vi "Test.vi"() -> ()   [LabVIEW 2018]
uses:
  <vilib>/Platform/TimedLoop/XDataNode/timing_clust.ctl
  <vilib>/Platform/TimedLoop/XDataNode/nitl_modes.ctl
  <vilib>/Platform/TimedLoop/XDataNode/wakeup.ctl
  <vilib>/rvi/Emulation/niFpgaSctlEmulationGetInTimedLoop.vi
  <vilib>/rvi/Emulation/niFpgaEmulationReportErrorSimple.vi
  <vilib>/rvi/Emulation/niFpgaGetClockAttributes.vi
  <vilib>/rvi/Emulation/niFpgaCriticalErrorInLSC.vi
  <vilib>/rvi/eio/common/nirviEmuTemplateMethod_errors.vi
  <vilib>/Platform/TimedLoop/XDataNode/XDataNode.xnode
  <vilib>/eio/EIONode/EIONode.xnode
  <vilib>/Platform/TimedLoop/XDataNode/XDNodeRunTimeDep.lvlib
panel:
  out "Record":i16[](array[numeric])
  out "Round":u64 format="%.0e"
  out "Out":bool
  out "Test":bool
  out "2V":bool
  out "2H":bool
  out "1V":bool
  out "1H":bool
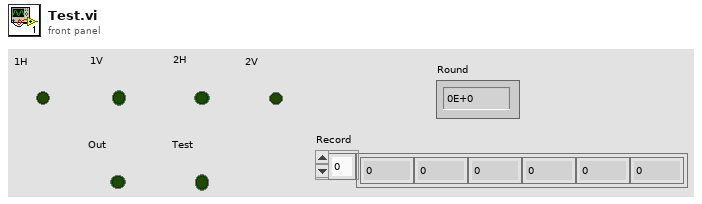
[diagram p1: front panel]
types:
  T1 = typedef "XDNodeRunTimeDep.lvlib/timing_clust.ctl" = cluster{"Expected End [f-1]":u64, "Actual End [f-1]":u64, "Finished Late? [f-1]":bool, "Expected End [i-1]":u64, "Actual End [i-1]":u64, "Finished Late? [i-1]":bool, "Expected Start [i]":u64, "Actual Start [i]":u64, "Expected Start [f]":u64, "Actual Start [f]":u64, "Source Name":string, "Structure Name":string, "Period":i64, "Deadline":i64, "Offset":i64, "Start":i64, "Priority":i32, "Timeout":i32, "Mode":T2, "Wakeup Reason":T3, "Error":errorcluster, "Source Type":string, "Secondary Source Type":string, "Global End Time":u64, "Global Start Time":u64, "Frame Duration":u64, "Iteration Duration":u64, "Assigned CPU":i32, "I/O Scan Engine Mode":u32}
  T2 = typedef "XDNodeRunTimeDep.lvlib/nitl_modes.ctl" = enum32{"No Change", "Process missed periods, maintain original phase", "Discard missed periods, maintain original phase", "Process missed periods, ignore original phase", "Discard missed periods, ignore original phase"}
  T3 = typedef "XDNodeRunTimeDep.lvlib/wakeup.ctl" = enum32{"Normal", "Aborted", "Asynchronous wakeup", "Timing source error", "Timed loop error", "Timeout"}
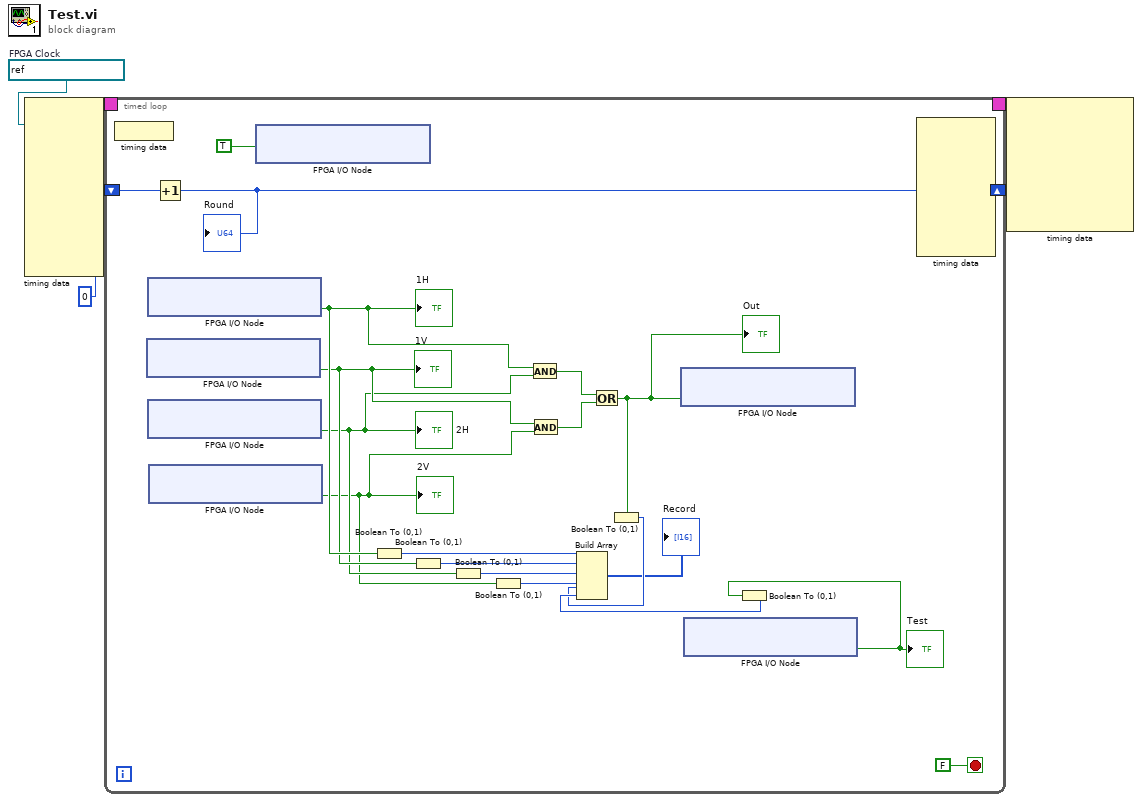
[diagram p0: block diagram]
diagram:
  w2 = refnum<k21> "200 MHz Clock"  # FPGA Clock
  n1 = node-c288(w2) -> (w4:T1)  [unwired: 9 in]
  n2 = timed-loop {
    timing: w4 -> [_]
    timing-out: [_] -> w3
    shift-right: [w18] -> _
    shift-left: i16 0 -> [w19]
    stop <- FALSE stop-if-true
    n3 = node-c288() -> ()  [unwired: 1 in]
    n4 = xnode "FPGA I/O Node"() -> ("IO Module\\SE_Ch2_Rd"=w14:bool)  [unwired: 1 in, 1 out]
    "1V" <- w14
    n5 = xnode "FPGA I/O Node"() -> ("IO Module\\SE_Ch1_Rd"=w17:bool)  [unwired: 1 in, 1 out]
    "1H" <- w17
    n6 = xnode "FPGA I/O Node"() -> ("IO Module\\SE_Ch3_Rd"=w12:bool)  [unwired: 1 in, 1 out]
    "2H" <- w12
    n7 = xnode "FPGA I/O Node"() -> ("IO Module\\SE_Ch4_Rd"=w7:bool)  [unwired: 1 in, 1 out]
    "2V" <- w7
    n8 = Increment(x=w19) -> (x+1=w18:i16)
    "Round" <- w18
    n9 = xnode "FPGA I/O Node"("IO Module\\SE_Ch5_Dir"=TRUE) -> ()  [unwired: 1 in, 1 out]
    n10 = Boolean To (0,1)(Boolean=w17) -> (0, 1=w16:i16)
    n11 = Boolean To (0,1)(Boolean=w14) -> (0, 1=w13:i16)
    n12 = Boolean To (0,1)(Boolean=w12) -> (0, 1=w11:i16)
    n13 = Boolean To (0,1)(Boolean=w7) -> (0, 1=w8:i16)
    n14 = And(x=w17, y=w12) -> (x .and. y?=w22:bool)
    n15 = And(x=w14, y=w7) -> (x .and. y?=w21:bool)
    n16 = Or(x=w22, y=w21) -> (x .or. y?=w15:bool)
    "Out" <- w15
    n17 = Boolean To (0,1)(Boolean=w15) -> (0, 1=w6:i16)
    n18 = xnode "FPGA I/O Node"("IO Module\\SE_Ch5_Wr"=w15) -> ()  [unwired: 1 in, 1 out]
    n19 = xnode "FPGA I/O Node"() -> ("IO Module\\SE_Ch6_Rd"=w10:bool)  [unwired: 1 in, 1 out]
    "Test" <- w10
    n20 = Boolean To (0,1)(Boolean=w10) -> (0, 1=w9:i16)
    n21 = Build Array(w16, w13, w11, w8, w6, w9) -> (→"Record":i16[])
    n22 = node-c288() -> ()  [unwired: 8 in, 1 out]
  }
  n23 = node-c288(w3) -> ()  [unwired: 7 out]
